vi "getDeviceName.vi"(8 "error in":errorcluster, 11 "connection ID in":refnum<k5>) -> (0 "error out":errorcluster, 2 "Device Name out":string, 3 "connection ID out":refnum<k5>)   [LabVIEW 2015]
panel:
  in  "Get Command":string="com.attocube.system.getDeviceName"
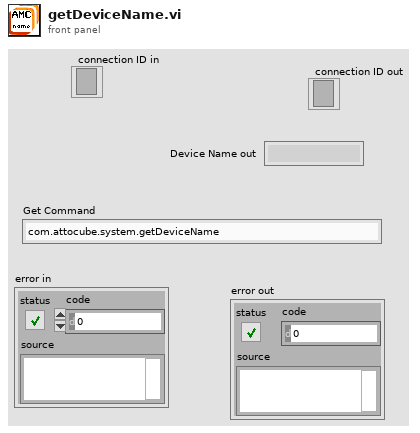
[diagram p1: front panel]
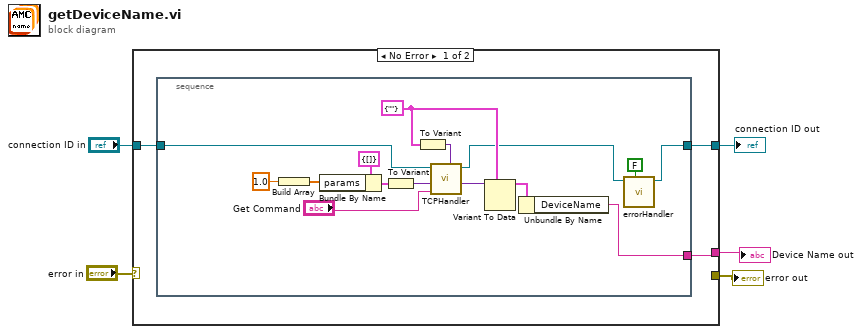
[diagram p0: block diagram]
diagram:
  n1 = case shown="No Error" "error in" {
    selector: "error in" -> [_ w25]
    tunnel: [_ w25] -> w5
    tunnel: "connection ID in" -> [w6 w24]
    tunnel: [w8 w24] -> w3
    tunnel: [w7 _] -> w1
    frame No Error {
      n2 = stacked-sequence {
        tunnel: [w9] -> w8
        tunnel: w6 -> [w16]
        tunnel: [w13] -> w7
        frame #0 {
          w14 = cluster{"DeviceName":string} {"DeviceName"=""} ("input cluster")
          n3 = Build Array(1.0 ("element")) -> (w20:dbl[])
          n4 = Bundle By Name(cluster=cluster{"params":i16[]} {"params"=[]} ("input cluster"), "params"=w20) -> (w21:cluster{"params":i16[]})
          n5 = To Variant(anything=w21) -> (Variant=w22:variant)
          n6 = To Variant(anything=w14) -> (Variant=w15:variant)
          n7 = call "TCPHandler.vi"("result Types"=w15, "method"="Get Command", "params"=w22, "connection ID"=w16) -> ("result"=w18:variant, "connection ID"=w10:refnum<k5>)  [unwired: 5 in, 1 out]
          n8 = Variant To Data(type=w14, Variant=w18) -> (data=w23:cluster{"DeviceName":string})  [unwired: 1 in, 1 out]
          n9 = Unbundle By Name(w23) -> ("DeviceName"=w13:string)
          n10 = call "errorHandler.vi"("show popup"=FALSE, "connection ID"=w10) -> ("connection ID"=w9:refnum<k5>)  [unwired: 8 in, 1 out]
        }
      }
    }
    frame Error {
    }
  }
  "error out" <- w5
  "Device Name out" <- w1
  "connection ID out" <- w3
